vi "Dashboard Main.vi"() -> ()   [LabVIEW 2012]
uses:
  <vilib>/event_ctls.llb/eventvkey.ctl
  <vilib>/Utility/config.llb/Read Key (String).vi
  <vilib>/Utility/config.llb/Read Key (I32).vi
  <vilib>/Utility/config.llb/Write Key (String).vi
  <vilib>/Utility/config.llb/Write Key (I32).vi
  <vilib>/Utility/config.llb/NI_LVConfig.lvlib
panel:
  in  "Camera Enable":bool
  in  "Camera Settings":T1={"Frate Rate"=30, "Compression"=30, "Size"=1} {"Frate Rate" scale=1.0..30.0; "Size" items=["640x480", "320x240", "160x120"]}
  out "Mode":T2(ring)=enum."Auto Disabled"
  out "Camera IP":string
  in  "Dashboard Tab":T3(tab)
  out "Desired Elevation":dbl(slide) scale=0.0..46.0
  out "Compressor Status":bool
  out "Manual RPM":dbl
  in  "Auto Fling":bool
  in  "Auto Spin":bool=TRUE
  in  "Auto Tilt":bool=TRUE
  out "Current Elevation":dbl(slide) scale=0.0..46.0
  out "At Speed":bool
  out "Spin":cluster{dbl, dbl}(knob) scale=0.0..5000.0
  out "Prespin":cluster{dbl, dbl}(knob) scale=0.0..5000.0
  in  "Set Front Pyramid Angle":bool
  in  "Set Feeder Station Preset":bool
  in  "Set Auton Shooter Speed":bool
  in  "Set Rear Pyramid Angle":bool
  in  "Set Behind Pyramid Angle":bool
  in  "Record Autonomous":bool
  in  "DB Camera Config":bool
  out "Mbps":dbl format="%#.1g"
  out "Mbps 2":bool
  out "fps":dbl format="%#.1g"
  in  "Calibrate Arm Top":bool
  in  "Calibrate Arm Bottom":bool
  out "JS1 Z":dbl(slide) scale=-1.0..1.0 scale format="%#_2e"
  out "JS2 Z":dbl(slide) scale=-1.0..1.0 scale format="%#_2e"
  out "Joystick 1":cluster{"X":dbl, "Y":dbl}[](graph)
  out "Joystick 2":cluster{"X":dbl, "Y":dbl}[](graph)
  out "JS Buttons 1":T4
  out "JS Buttons 2":T4
  out "MotorSlide4":dbl(slide) scale=-1.0..1.0 scale format="%#_2e"
  out "MotorSlide3":dbl(slide) scale=-1.0..1.0 scale format="%#_2e"
  out "MotorSlide2":dbl(slide) scale=-1.0..1.0 scale format="%#_2e"
  in  "MotorName3":string="Front Left"
  in  "MotorName4":string="Front Right"
  in  "MotorName1":string="Rear Left"
  in  "MotorName2":string="Rear Right"
  out "MotorChart4":dbl(graph)
  out "MotorChart3":dbl(graph)
  out "MotorChart2":dbl(graph)
  out "MotorSlide1":dbl(slide) scale=-1.0..1.0 scale format="%#_2e"
  out "MotorChart1":dbl(graph)
  out "Battery Value":dbl(slide) scale=0.0..14.0 scale format="%#_2e"
  out "Battery":sgl(graph)
  out "Robot IP":string
  in  "Slider":dbl(slide) scale=0.0..100.0 scale format="%#_3g"
  in  "On/Off":bool caption="Solenoid"
  in  "Test Name":u16(ring) items=["Select the test to run...", "Example Test", "-------------------------------", "List of tests is built in robot code.", "Replace with your own automated tests."]
  in  "Test Tree":string(tree)
  in  "Motor":cluster{"Value":dbl, "Enable":bool} {"Value" scale=-1.0..1.0 scale format="%#_3g"}
  out "Progress":T5 {"Test Progress" scale=0.0..100.0}
  in  "Rev/Fwd":cluster{"Forward":bool, "Reverse":bool}
  in  "Ring":u16(ring) items=["Auto", "Fixed indoor", "Fixed outdoor 1", "Fixed outdoor 2", "Fixed fluorescent 1", "Fixed fluorescent 2", "Hold current"]
  in  "Listbox":i32(listbox)
  in  "Viewer":enum32{"Camera Image", "Variables"}(tab)
  out "Image Error Message":string="Timeout in Camera Communications"
  out "Camera Image":T6(plugin-control)
  out "Tree":string(tree)
  # "Drive & Motors"
  # "Robot IP:"
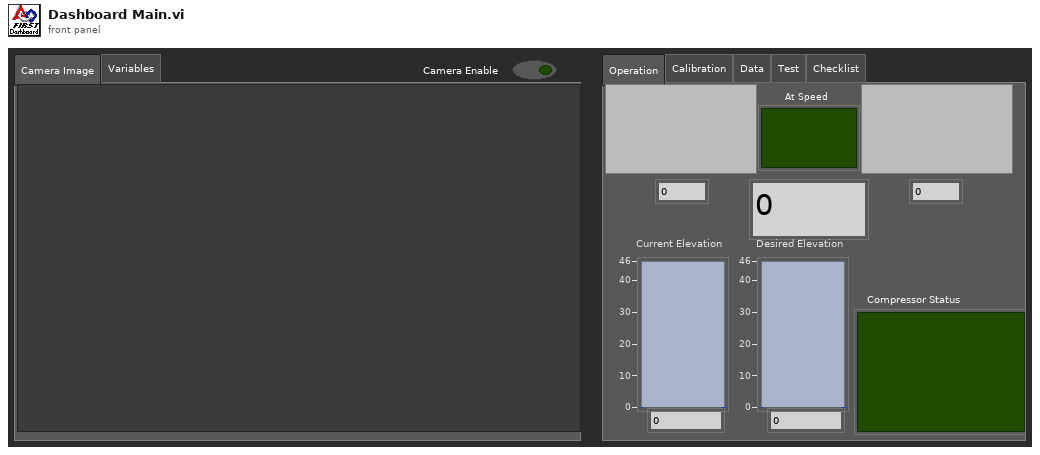
[diagram p1: front panel]
types:
  T1 = cluster{"Frate Rate":i32, "Compression":i32, "Size":u16}
  T2 = enum8{"Tele-Op Disabled", "Tele-Op Enabled", "Auto Disabled", "Auto Enabled", "Test Disabled", "Test Enabled", ""}
  T3 = enum32{"Operation", "Calibration", "Data", "Test", "Checklist"}
  T4 = cluster{bool, bool, bool, bool, bool, bool, bool, bool, bool, bool, bool, bool}
  T5 = cluster{"Test Progress":u8, "Test Progress Text":string}
  T6 = typedef "IMAQ Image.ctl" = refnum<image>
  T7 = typedef "Image Type" = u32
  T8 = typedef "SkeletonTrackState.ctl" = enum32{"NotTracked", "PositionOnly", "Tracked"}
  T9 = cluster{"TrackingState":u8[], "Position":cluster{"x":sgl, "y":sgl, "z":sgl}, cluster{"x":sgl, "y":sgl, "z":sgl, sgl}[], "TrackState":T8}
  T10 = cluster{cluster{"ScaledToPercentRange":dbl, "ScaledToPercentRange":dbl, "ScaledToPercentRange":dbl}, cluster{bool, bool, bool}}[]
  T11 = cluster{cluster{"ScaledToPercentRange":dbl, "ScaledToPercentRange":dbl, "ScaledToPercentRange":dbl}, cluster{bool, bool, bool}}
  T12 = typedef "LVRectTypeDef.ctl" = cluster{"Left":i16, "Top":i16, "Right":i16, "Bottom":i16}
  T13 = cluster{"Competition mode":bool, "Robot Link":bool, "Autonomous":bool, "Enabled":bool, "E-Stop":bool, "Simulated":bool, "TestMode":bool, "Docked Window":bool}
  T14 = cluster{"Boolean Array[0]":bool, "Boolean Array[1]":bool, "Boolean Array[2]":bool, "Boolean Array[3]":bool, "Boolean Array[4]":bool, "Boolean Array[5]":bool, "Boolean Array[6]":bool, "Boolean Array[7]":bool, "Boolean Array[8]":bool, "Boolean Array[9]":bool, "Boolean Array[10]":bool, "Boolean Array[11]":bool}
  T15 = typedef "NI_LVConfig.lvlib/Config Data RefNum.ctl" = refnum<k1>
  T16 = typedef "eventvkey.ctl" = enum16{"ASCII", "Enter", "Return", "Shift", "Ctrl", "Alt", "Cmd", "Opt", "Caps", "NumLock", "Clear", "Break", "Up", "Down", "Left", "Right", "Insert", "Delete", "Home", "End", "PageUp", "PageDown", "Escape", "Help", "Pause", "ScrollLock", "F1", "F2", "F3", "F4", "F5", "F6", "F7", "F8", "F9", "F10", "F11", "F12", "F13", "F14", "F15", "F16", "F17", "F18", "F19", "F20", "F21", "F22", "F23", "F24", "Play", "VolumeUp", "VolumeDown", "Mute", "Two Byte Char"}
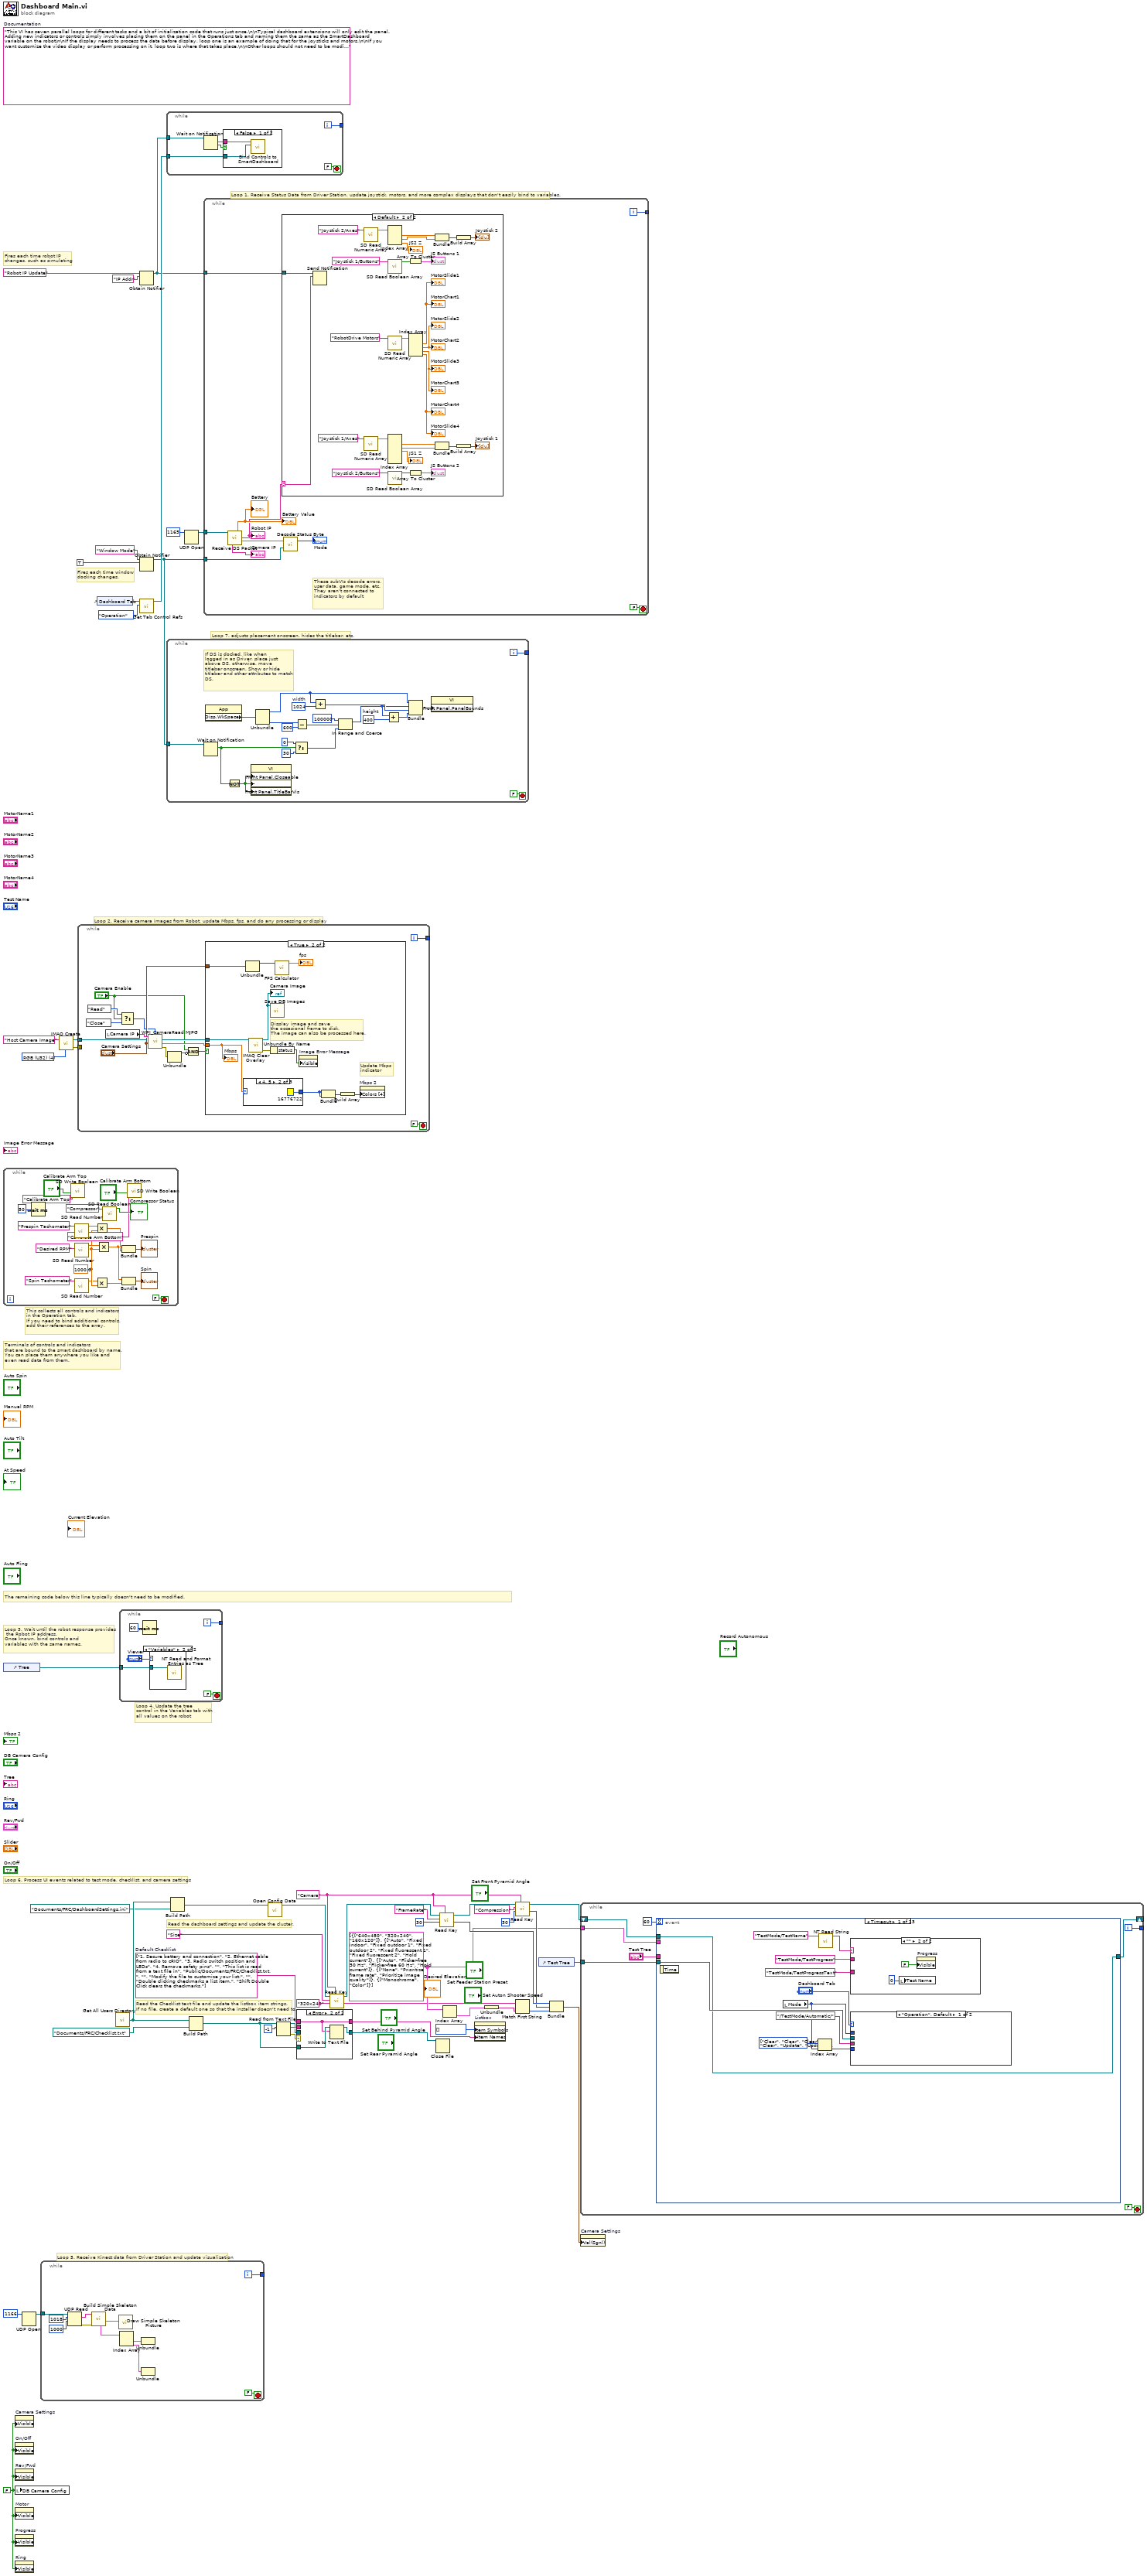
[diagram p0: block diagram]
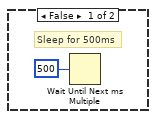
[diagram p3: hidden frame]
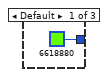
[diagram p4: hidden frame]
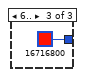
[diagram p5: hidden frame]
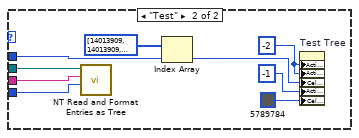
[diagram p7: hidden frame]
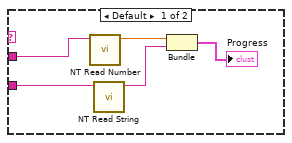
[diagram p8: hidden frame]
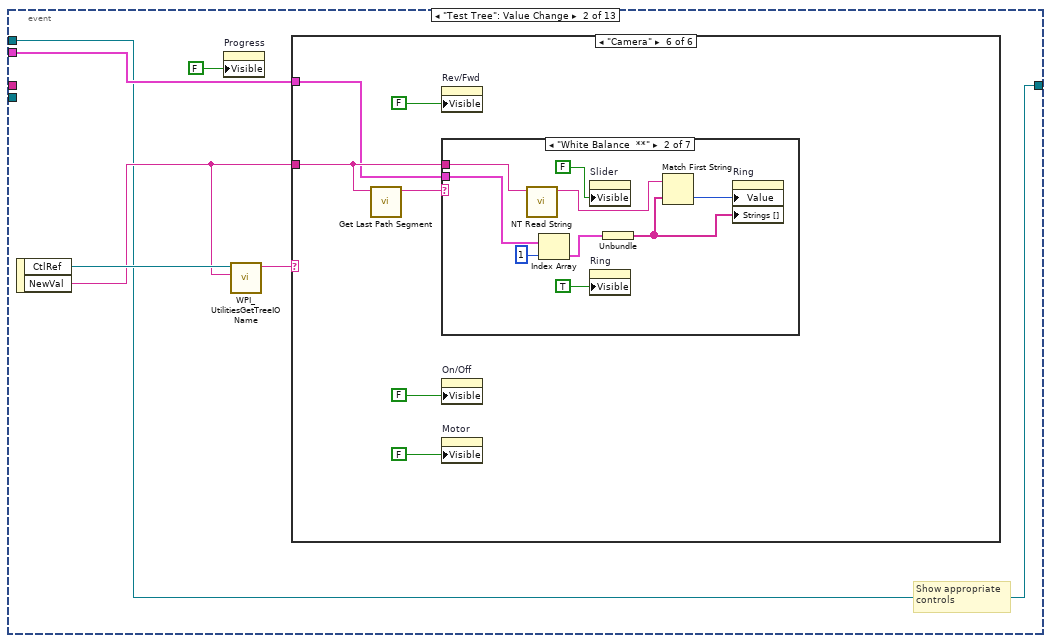
[diagram p9: hidden frame]
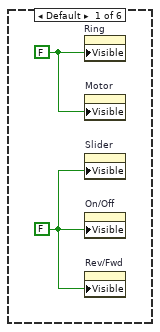
[diagram p10: hidden frame]
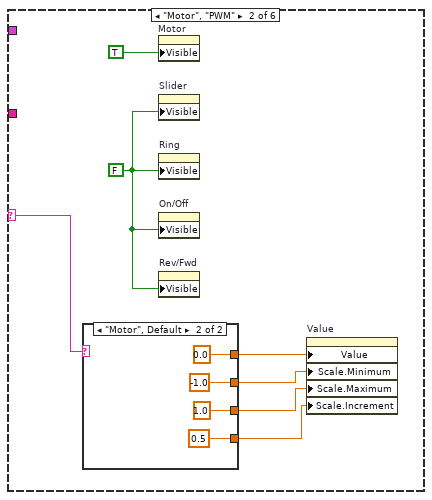
[diagram p11: hidden frame]
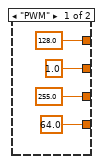
[diagram p12: hidden frame]
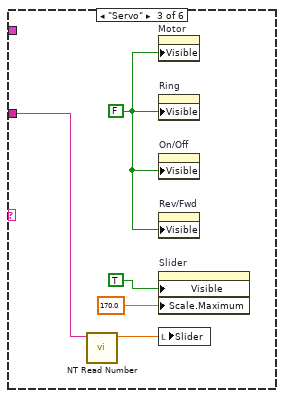
[diagram p13: hidden frame]
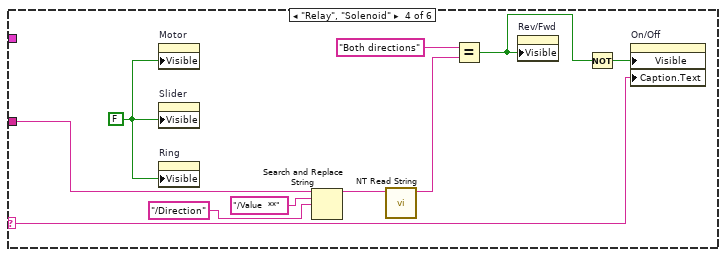
[diagram p14: hidden frame]
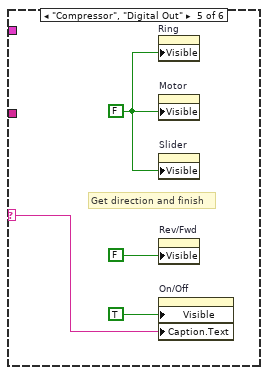
[diagram p15: hidden frame]
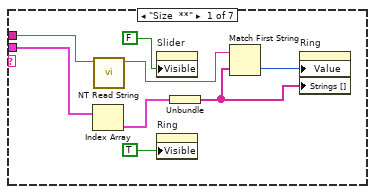
[diagram p16: hidden frame]
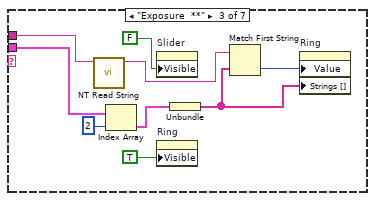
[diagram p17: hidden frame]
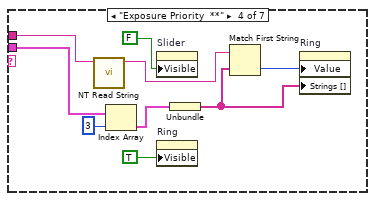
[diagram p18: hidden frame]
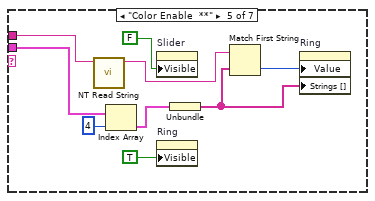
[diagram p19: hidden frame]
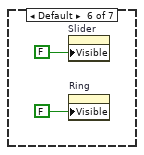
[diagram p20: hidden frame]
diagram:
  w21 = "Camera"
  w13 = cluster{string[]}[] [{["640x480", "320x240", "160x120"]}, {["Auto", "Fixed indoor", "Fixed outdoor 1", "Fixed outdoor 2", "Fixed fluorescent 1", "Fixed fluorescent 2", "Hold current"]}, {["Auto", "Flicker-free 50 Hz", "Flicker-free 60 Hz", "Hold current"]}, {["None", "Prioritize frame rate", "Prioritize image quality"]}, {["Monochrome", "Color"]}]
  w29 = string[] ["1. Secure battery and connection", "2. Ethernet cable from radio to cRIO", "3. Radio switch position and LEDs", "4. Remove safety pins", "", "This list is read from a text file in", "Public/Documents/FRC/Checklist.txt.", "", "Modify the file to customize your list.", "", "Double clicking checkmarks a list item.", "Shift Double Click clears the checkmarks."]  # Default Checklist
  w27 = FALSE ("Visible")
  (unwired) "This VI has seven parallel loops for different tasks and a bit of initialization code that runs just once.\n\nTypical dashboard extensions will only edit the panel. Adding new indicators or controls simply involves placing them on the panel in the Operations tab and naming them the same as the SmartDashboard variable on the robot\n\nIf the display needs to process the data before display, loop one is an example of doing that for the joysticks and motors.\n\nIf you want customize the video display or perform processing on it, loop two is where that takes place.\n\nOther loops should not need to be modified. They are pretty standard, and document the task they perform."  # Documentation
  w50 = T7 4 items=["Grayscale (U8)", "Grayscale (I16)", "Grayscale (SGL)", "Complex (CSG)", "RGB (U32)", "HSL (U32)", "RGB (U64)"] ("Image Type")
  # "Fires each time robot IP\nchanges, such as simulating"
  # "Fires each time window\ndocking changes."
  # "Read the Checklist text file and update the listbox item strings.\nIf no file, create a default one so that the installer doesn't need to."
  # "This collects all controls and indicators\nin the Operation tab.\nIf you need to bind additional controls,\nadd their references to the array."
  # "The remaining code below this line typically doesn't need to be modified."
  # "Loop 6. Process UI events related to test mode, checklist, and camera settings"
  # "Read the dashboard settings and update the cluster."
  # "Terminals of controls and indicators\nthat are bound to the smart dashboard by name.\nYou can place them anywhere you like and\neven read data from them."
  # "Loop 4. Update the tree\ncontrol in the Variables tab with\nall values on the robot"
  # "Loop 3. Wait until the robot response provides\n the Robot IP address.\nOnce known, bind controls and\nvariables with the same names."
  # "Loop 5. Receive Kinect data from Driver Station and update visualization"
  # "Loop 7. adjusts placement onscreen, hides the titlebar, etc."
  # "Loop 1. Receive Status Data from Driver Station, update joystick, motors, and more complex displays that don't easily bind to variables."
  # "Loop 2. Receive camera images from Robot, update Mbps, fps, and do any processing or display"
  n1 = while {
    stop <- FALSE stop-if-true
    w65 = 1000.0 ("y")
    n2 = Wait (ms)(milliseconds to wait=u32 50) -> ()  [unwired: 1 out]
    n3 = call <vilib>:"SD Write Boolean.vi"("Boolean"="Calibrate Arm Top", "Name"="Calibrate Arm Top") -> ()  [unwired: 8 in, 2 out]
    n4 = call <vilib>:"SD Read Number.vi"("Name"="Prespin Tachometer") -> ("Numeric"=w64:dbl)  [unwired: 8 in, 2 out]
    n5 = call <vilib>:"SD Read Number.vi"("Table Prefix"="Desired RPM") -> ("Numeric"=w66:dbl)  [unwired: 8 in, 2 out]
    n6 = call <vilib>:"SD Read Number.vi"("Name"="Spin Tachometer") -> ("Numeric"=w62:dbl)  [unwired: 8 in, 2 out]
    n7 = Multiply(x=w64, y=w65) -> (x*y=w63:dbl)
    n8 = Multiply(x=w62, y=w65) -> (x*y=w61:dbl)
    n9 = Multiply(x=w66, y=w65) -> (x*y=w67:dbl)
    n10 = call <vilib>:"SD Read Boolean.vi"("Name"="Compressor") -> ("Boolean"=→"Compressor Status":bool)  [unwired: 8 in, 2 out]
    n11 = Bundle(w67, w63) -> (→"Prespin":cluster{dbl, dbl})  [unwired: 1 in]
    n12 = Bundle(w67, w61) -> (→"Spin":cluster{dbl, dbl})  [unwired: 1 in]
    n13 = call <vilib>:"SD Write Boolean.vi"("Boolean"="Calibrate Arm Bottom", "Name"="Calibrate Arm Bottom") -> ()  [unwired: 8 in, 2 out]
  }
  n14 = control-ref of="Tree"() -> (w2:refnum<vi>)
  n15 = property on="Camera Settings" class="Clust (strict)"("Visible"=w27) -> ()  [unwired: 2 in, 2 out]
  n16 = property on="On/Off" class="Bool (strict)"("Visible"=w27) -> ()  [unwired: 2 in, 2 out]
  n17 = property on="Rev/Fwd" class="Clust (strict)"("Visible"=w27) -> ()  [unwired: 2 in, 2 out]
  n18 = local write "DB Camera Config"(w27) -> ()
  n19 = property on="Motor" class="Clust (strict)"("Visible"=w27) -> ()  [unwired: 2 in, 2 out]
  n20 = property on="Progress" class="Clust (strict)"("Visible"=w27) -> ()  [unwired: 2 in, 2 out]
  n21 = property on="Ring" class="Ring (strict)"("Visible"=w27) -> ()  [unwired: 2 in, 2 out]
  n22 = UDP Open(11:u16 1166 ("port")) -> (port=w45:refnum<k16>)  [unwired: 2 in, 4 out]
  n23 = while {
    tunnel: w45 -> [w81]
    tunnel: [w74] -> _
    i -> [w74]
    stop <- FALSE stop-if-true
    n24 = UDP Read(connection ID=w81, max size (548)=1018 ("bytes to read"), timeout ms (25000)=1000) -> (data out=w79:string, error out=w73:errorcluster)  [unwired: 1 in, 3 out]
    n25 = call "Build Simple Skeleton Data.vi"("error in (no error)"=w73, "data in"=w79) -> ("Skeleton Data"=w80:T9, "Simple Joystick Info"=w77:T10)  [unwired: 5 in, 3 out]
    n26 = call "Draw Simple Skeleton Picture.vi"("Simple Skeleton"=w80) -> ()  [unwired: 10 in, 1 out]
    n27 = Index Array(array=w77) -> (element #1=w76:T11, element #2=w75:T11)  [unwired: 2 in]
    n28 = Unbundle(w76) -> ()  [unwired: 2 out]
    n29 = Unbundle(w75) -> ()  [unwired: 2 out]
  }
  n30 = call "IMAQ Create"("Image Name"="Host Camera Image", "Image Type"=w50) -> ("New Image"=w48:T6, "error out"=w47:errorcluster)  [unwired: 2 in, 1 out]
  n31 = while {
    tunnel: w48 -> [w93]
    tunnel: w47 -> [_]
    tunnel: [w96] -> _
    i -> [w96]
    stop <- FALSE stop-if-true
    n32 = local read "Camera IP"() -> (w95:string)
    n33 = Select(t=enum16{"Read", "Reopen", "Close"}."Read" ("Operation"), s="Camera Enable", f=enum16{"Read", "Reopen", "Close"}."Close" ("Operation")) -> (s? t:f=w88:enum16{"Read", "Reopen", "Close"})
    n34 = call <vilib>:"WPI_CameraRead MJPG.vi"("Operation"=w88, "Camera Settings"="Camera Settings", "Image"=w93, "address"=w95) -> ("error out"=w87:errorcluster, "Bandwidth (kbps)"=w91:dbl, "Image Out"=w92:T6)  [unwired: 5 in]
    n35 = Unbundle(w87) -> ("status"=w85:bool)  [unwired: 2 out]
    n36 = Compound Arithmetic op=AND("Camera Enable", invert w85) -> (w84:bool)
    n37 = case shown="True" w84 {
      tunnel: "Camera Settings" -> [_ w100]
      tunnel: w92 -> [_ w103]
      tunnel: w91 -> [_ w102]
      frame False {
        # "Sleep for 500ms"
        n38 = Wait Until Next ms Multiple(millisecond multiple=u32 500) -> ()  [unwired: 1 out]
      }
      frame True {
        # "Display image and save\nthe occasional frame to disk.\nThe image can also be processed here."
        # "Update Mbps\nindicator"
        n39 = case shown="4, 5" w102 {
          tunnel: [u32 6618880 ("Color Box") u32 16776722 ("Color Box") u32 16716800 ("Color Box")] -> w104
          frame Default {
          }
          frame 4, 5 {
          }
          frame 6.. {
          }
        }
        n40 = Unbundle(w100) -> ("Frate Rate"=w99:i32)  [unwired: 2 out]
        n41 = call "IMAQ Clear Overlay"("Image"=w103) -> ("error out"=w108:errorcluster, "Image Out"=w107:T6)  [unwired: 2 in, 7 out]
        "Camera Image" <- w107
        n42 = call "Save DB Images.vi"("Image"=w107) -> ()  [unwired: 2 in, 1 out]
        n43 = Unbundle By Name(w108) -> ("status"=w109:bool)
        n44 = call "FPS Calculator.vi"("Average Count"=w99) -> ("fps"=→"fps":dbl)  [unwired: 10 in]
        n45 = property on="Image Error Message" class="Str"("Visible"=w109) -> ()  [unwired: 2 in, 2 out]
        n46 = Bundle("Color Box"=w104, "Color Box"=w104) -> (w106:cluster{"Color Box":u32, "Color Box":u32})  [unwired: 1 out]
        n47 = Build Array(w106) -> (w105:cluster{"Color Box":u32, "Color Box":u32}[])
        n48 = property on="Mbps 2" class="Bool (strict)"("Colors [4]"=w105) -> ()  [unwired: 2 in, 2 out]
        "Mbps" <- w102
      }
    }
  }
  n49 = control-ref of="Dashboard Tab"() -> (w43:refnum<vi>)
  n50 = call "Get All Users Directory.vi"() -> ("All User Path"=w26:path)
  n51 = while {
    tunnel: [w114] -> _
    tunnel: w2 -> [w113]
    i -> [w114]
    stop <- FALSE stop-if-true
    n52 = Wait (ms)(milliseconds to wait=u32 60) -> ()  [unwired: 1 out]
    n53 = case shown="\"Variables\"" "Viewer" {
      tunnel: w113 -> [_ w118]
      frame Default {
      }
      frame "Variables" {
        n54 = call <vilib>:"NT Read and Format Entries as Tree.vi"("Tree Refnum"=w118) -> ()  [unwired: 9 in, 2 out]
      }
    }
  }
  n55 = Obtain Notifier(name (unnamed)="Robot IP Update", notification data type="IP Addr" ("name (unnamed)")) -> (notifier out=w40:refnum<notifier>)  [unwired: 2 in, 2 out]
  n56 = Obtain Notifier(name (unnamed)="Window Mode", notification data type=TRUE) -> (notifier out=w33:refnum<notifier>)  [unwired: 2 in, 2 out]
  n57 = call <vilib>:"Get Tab Control Refs.vi"("Page Index"=enum32{"Operation", "Test"}."Operation" ("Dashboard Tab"), "TabControl in"=w43) -> ("ControlsOnPage"=w44:refnum<vi>[])  [unwired: 9 in]
  n58 = while {
    tunnel: w44 -> [w124]
    tunnel: w40 -> [w121]
    tunnel: [w119] -> _
    i -> [w119]
    stop <- FALSE stop-if-true
    n59 = Wait on Notification(notifier=w121) -> (notification=w120:string, timed out?=w122:bool)  [unwired: 3 in, 2 out]
    n60 = case shown="False" w122 {
      tunnel: w124 -> [w126 _]
      tunnel: w120 -> [w125 _]
      frame False {
        n61 = call <vilib>:"Bind Controls to SmartDashboard.vi"("Bound Control Refs"=w126, "Server IP Address"=w125) -> ()  [unwired: 10 in]
      }
      frame True {
      }
    }
  }
  n62 = while {
    tunnel: w33 -> [w145]
    tunnel: [w143] -> _
    i -> [w143]
    stop <- FALSE stop-if-true
    w135 = 1024  # width
    w138 = 400  # height
    # "If DS is docked, like when\nlogged in as Driver, place just\nabove DS, otherwise, move\ntitlebar onscreen. Show or hide\ntitlebar and other attributes to match\nDS."
    n63 = Wait on Notification(notifier=w145) -> (notification=w130:bool)  [unwired: 3 in, 3 out]
    n64 = property class="App"() -> ("Disp.WkSpace"=w141:T12)  [unwired: 2 in, 2 out]
    n65 = Not(x=w130) -> (.not. x?=w144:bool)
    n66 = property class="VI"("Front Panel.Closeable"=w144, "Front Panel.Minimizeable"=w144, "Front Panel.TitleBarVis"=w144) -> ()  [unwired: 2 in, 2 out]
    n67 = Unbundle(w141) -> ("Left"=w139:i16, "Bottom"=w136:i16)  [unwired: 2 out]
    n68 = Select(t=0, s=w130, f=30) -> (s? t:f=w129:i32)
    n69 = Subtract(x=w136, y=600) -> (x-y=w133:i32)
    n70 = Add(x=w139, y=w135) -> (x+y=w140:i32)
    n71 = In Range and Coerce(upper limit=100000, x=w133, lower limit=w129) -> (coerced(x)=w127:i32)  [unwired: 1 out]
    n72 = Add(x=w127, y=w138) -> (x+y=w137:i32)
    n73 = Bundle("Left"=w139, w127, w140, w137) -> (w142:cluster{"Left":i16, i32, i32, i32})  [unwired: 1 out]
    n74 = property class="VI"("Front Panel.PanelBounds"=w142) -> ()  [unwired: 2 in, 2 out]
  }
  n75 = Build Path(base path=w26, name or relative path=path "Documents/FRC/DashboardSettings.ini") -> (appended path=w25:path)
  n76 = UDP Open(11:u16 1165 ("port")) -> (port=w51:refnum<k16>)  [unwired: 2 in, 4 out]
  n77 = Build Path(base path=w26, name or relative path=path "Documents/FRC/Checklist.txt") -> (appended path=w30:path)
  n78 = while {
    tunnel: w51 -> [w154]
    tunnel: w40 -> [w148]
    tunnel: w33 -> [w152]
    tunnel: [w149] -> _
    i -> [w149]
    stop <- FALSE stop-if-true
    # "These subVIs decode errors, user data, game mode, etc.\nThey aren't connected to indicators by default"
    n79 = call "Receive DS Packet.vi"("Recv Socket"=w154) -> ("Battery"=→"Battery" →"Battery Value":sgl, "Robot IP Address"=w147:string, "Status"=w155:T13, "Camera IP Address"=→"Camera IP":string)  [unwired: 1 in, 10 out]
    "Robot IP" <- w147
    n80 = case shown="Default" w147 {
      selector: w147 -> [_ w157]
      tunnel: w148 -> [_ w158]
      frame "0.0.0.0" {
        # "Robot not responding, don't poll the variables"
      }
      frame Default {
        n81 = Send Notification(notification=w157, notifier=w158) -> ()  [unwired: 1 in, 2 out]
        n82 = call <vilib>:"SD Read Numeric Array.vi"("Name"="Joystick 2/Axes") -> ("Numeric Array"=w168:dbl[])  [unwired: 8 in, 2 out]
        n83 = call <vilib>:"SD Read Numeric Array.vi"("Name"="Joystick 1/Axes") -> ("Numeric Array"=w174:dbl[])  [unwired: 8 in, 2 out]
        n84 = Index Array(array=w168) -> (element #1=w163:dbl, element #2=w162:dbl, element #3=→"JS2 Z":dbl)  [unwired: 3 in]
        n85 = call <vilib>:"SD Read Boolean Array.vi"("Name"="Joystick 1/Buttons") -> ("Boolean Array"=w176:bool[])  [unwired: 8 in, 2 out]
        n86 = call <vilib>:"SD Read Numeric Array.vi"("Name"="RobotDrive Motors") -> ("Numeric Array"=w181:dbl[])  [unwired: 8 in, 2 out]
        n87 = Index Array(array=w174) -> (element #1=w171:dbl, element #2=w172:dbl, element #3=→"JS1 Z":dbl)  [unwired: 6 in, 3 out]
        n88 = call <vilib>:"SD Read Boolean Array.vi"("Name"="Joystick 2/Buttons") -> ("Boolean Array"=w167:bool[])  [unwired: 8 in, 2 out]
        n89 = Array To Cluster(array=w176) -> (cluster=→"JS Buttons 1":T14)
        n90 = Array To Cluster(array=w167) -> (cluster=→"JS Buttons 2":T14)
        n91 = Index Array(array=w181) -> (element #1=→"MotorChart1" →"MotorSlide1":dbl, element #2=→"MotorSlide2" →"MotorChart2":dbl, element #3=→"MotorChart3" →"MotorSlide3":dbl, element #4=→"MotorChart4" →"MotorSlide4":dbl)  [unwired: 4 in]
        n92 = Bundle("Numeric"=w163, "Numeric"=w162) -> (w164:cluster{"Numeric":dbl, "Numeric":dbl})  [unwired: 1 in]
        n93 = Bundle("Numeric"=w171, "Numeric"=w172) -> (w170:cluster{"Numeric":dbl, "Numeric":dbl})  [unwired: 1 in]
        n94 = Build Array(w164) -> (→"Joystick 2":cluster{"Numeric":dbl, "Numeric":dbl}[])
        n95 = Build Array(w170) -> (→"Joystick 1":cluster{"Numeric":dbl, "Numeric":dbl}[])
      }
    }
    n96 = call "Decode Status Byte.vi"("Window Mode Notifier"=w152, "Status"=w155) -> ("Mode"=→"Mode":T2)  [unwired: 1 out]
  }
  n97 = call <vilib>:"Open Config Data.vi"("configuration file path"=w25) -> ("refnum"=w24:T15)  [unwired: 8 in, 2 out]
  n98 = Read from Text File(file (use dialog)=w30, count=-1 ("timeout ms (25000)")) -> (refnum out=w8:refnum<file>, text=w31:string[], error out=w32:errorcluster)  [unwired: 2 in, 1 out]
  n99 = case shown="Error" w32 {
    tunnel: w31 -> [w186 _]
    tunnel: [w186 w188] -> w28
    tunnel: w29 -> [_ w188]
    tunnel: w30 -> [_ w189]
    tunnel: [w185 w187] -> w7
    tunnel: w8 -> [w185 _]
    frame No Error {
    }
    frame Error {
      n100 = Write to Text File(file (use dialog)=w189, text=w188) -> (refnum out=w187:refnum<file>)  [unwired: 2 in, 2 out]
    }
  }
  n101 = call-poly <vilib>:"Read Key.vi"("section"=w21, "default value"="320x240", "key"="Size", "refnum"=w24) -> ("value"=w11:string, "refnum out"=w6:T15)  [unwired: 2 in, 4 out]
  n102 = Close File(refnum=w7) -> ()  [unwired: 1 in, 2 out]
  n103 = call-poly <vilib>:"Read Key.vi"("section"=w21, "default value"=30, "key"="FrameRate", "refnum"=w6) -> ("value"=w16:i32, "refnum out"=w5:T15)  [unwired: 1 in, 5 out]
  n104 = Index Array(array=w13) -> (element=w14:cluster{string[]})  [unwired: 1 in]
  n105 = property on="Listbox" class="LstBox (strict)"("Item Symbols"=i32[] [], "Item Names"=w28) -> ()  [unwired: 2 in, 2 out]
  n106 = Unbundle(w14) -> (w12:string[])
  n107 = call-poly <vilib>:"Read Key.vi"("section"=w21, "default value"=30, "key"="Compression", "refnum"=w5) -> ("value"=w15:i32, "refnum out"=w3:T15)  [unwired: 1 in, 5 out]
  n108 = Match First String(2:w12, 3:w11) -> (0:w10:i32)  [unwired: 1 out]
  n109 = control-ref of="Test Tree"() -> (w1:refnum<vi>)
  n110 = Bundle("value"=w16, "value"=w15, "index"=w10) -> (w4:cluster{"value":i32, "value":i32, "index":i32})  [unwired: 1 out]
  n111 = while {
    tunnel: w13 -> [w194]
    shift-right: [w193] -> _
    shift-left: w3 -> [w192]
    tunnel: [w191] -> _
    tunnel: w1 -> [w190]
    i -> [w191]
    stop <- FALSE stop-if-true
    n112 = event shown="[0] Timeout" {
      selector: _ -> [_ _ _ _ _ _ _ _ _ _ _ _ _]
      dyn-events: _ -> [_ _ _ _ _ _ _ _ _ _ _ _ _]
      timeout: u32 60 ("milliseconds to wait") -> [_ _ _ _ _ _ _ _ _ _ _ _ _]
      tunnel: w190 -> [w204 _ _ _ _ _ _ _ _ _ _ _ _]
      tunnel: "Test Tree" -> [_ _ _ _ _ _ _ _ w398 w406 w408 w412 w420]
      tunnel: w194 -> [_ w226 _ _ _ _ w362 w392 _ _ _ _ _]
      tunnel: [w198 w225 _ w328 w336 w348 w361 w385 w397 w404 w407 w411 w419] -> w193
      tunnel: w192 -> [w198 w225 _ w328 w336 w348 w360 w385 w397 w404 w407 w411 w419]
      event Timeout {
        w203 = enum16{"Update", "Clear"}[] [enum."Clear", enum."Clear", enum."Clear", enum."Clear", enum."Update", enum."Update", enum."Clear"] items=["Update", "Clear"]
        n113 = event-data() -> ()  [unwired: 1 in, 1 out]
        n114 = local read "Mode"() -> (w201:T2)
        n115 = Index Array(array=w203, index=w201) -> (element=w202:enum16{"Update", "Clear"})
        n116 = call <vilib>:"NT Read String.vi"("Name"="TestMode/TestName") -> ("String"=w207:string)  [unwired: 9 in, 1 out]
        n117 = case shown="\"\"" w207 {
          tunnel: "TestMode/TestProgress" ("Name") -> [w219 _]
          tunnel: "TestMode/TestProgressText" ("Name") -> [w218 _]
          frame Default {
            n118 = call <vilib>:"NT Read Number.vi"("Name"=w219) -> ("Numeric"=w220:dbl)  [unwired: 9 in, 1 out]
            n119 = call <vilib>:"NT Read String.vi"("Name"=w218) -> ("String"=w221:string)  [unwired: 9 in, 1 out]
            n120 = Bundle("Numeric"=w220, "String"=w221) -> (→"Progress":cluster{"Numeric":dbl, "String":string})  [unwired: 1 in]
          }
          frame "" {
            n121 = local write "Test Name"(u16 0) -> ()
            n122 = property on="Progress" class="Clust (strict)"("Visible"=FALSE) -> ()  [unwired: 2 in, 2 out]
          }
        }
        n123 = case shown="\"Operation\", Default" "Dashboard Tab" {
          tunnel: w204 -> [_ w217]
          tunnel: "/TestMode/Automatic/" ("Name Pattern") -> [_ w216]
          tunnel: w202 -> [_ w215]
          tunnel: w201 -> [_ w213]
          frame "Operation", Default {
          }
          frame "Test" {
            w212 = -2 ("Active Item:Row Number")
            n124 = call <vilib>:"NT Read and Format Entries as Tree.vi"("Operation"=w215, "Name Pattern"=w216, "Tree Refnum"=w217) -> ()  [unwired: 7 in, 2 out]
            n125 = Index Array(array=u32[] [14013909, 14013909, 14013909, 14013909, 14013909, 16777215, 14013909], index=w213) -> (element=w211:u32)
            n126 = property on="Test Tree" class="Tree (strict)"("Active Item Row Number"=w212, "ActiveColNum"=w212, "CellBG"=w211, "Active Item Row Number"=-1 ("Active Item:Row Number"), "CellBG"=u32 5789784 ("Color Box")) -> ()  [unwired: 2 in, 2 out]
          }
        }
      }
      event "Test Tree": Value Change {
        # "Show appropriate\ncontrols"
        n127 = event-data() -> ("CtlRef"=w229:refnum<vi>, "NewVal"=w227:string)  [unwired: 1 in]
        n128 = property on="Progress" class="Clust (strict)"("Visible"=FALSE) -> ()  [unwired: 2 in, 2 out]
        n129 = call <vilib>:"WPI_UtilitiesGetTreeIOName.vi"("NewVal"=w227, "TreeControl in"=w229) -> ("I/O Name"=w230:string)  [unwired: 9 in]
        n130 = case shown="\"Camera\"" w230 {
          selector: w230 -> [_ w237 _ w255 w264 _]
          tunnel: w227 -> [_ _ w252 w254 _ w271]
          tunnel: w226 -> [_ _ _ _ _ w270]
          frame Default {
            w232 = FALSE ("Visible")
            w231 = FALSE ("Visible")
            n131 = property on="Ring" class="Ring (strict)"("Visible"=w231) -> ()  [unwired: 2 in, 2 out]
            n132 = property on="Motor" class="Clust (strict)"("Visible"=w231) -> ()  [unwired: 2 in, 2 out]
            n133 = property on="Slider" class="Slide (strict)"("Visible"=w232) -> ()  [unwired: 2 in, 2 out]
            n134 = property on="On/Off" class="Bool (strict)"("Visible"=w232) -> ()  [unwired: 2 in, 2 out]
            n135 = property on="Rev/Fwd" class="Clust (strict)"("Visible"=w232) -> ()  [unwired: 2 in, 2 out]
          }
          frame "Motor", "PWM" {
            w238 = FALSE ("Visible")
            n136 = case shown="\"Motor\", Default" w237 {
              tunnel: [1.0 ("Value") -1.0 ("Value")] -> w236
              tunnel: [255.0 ("Value") 1.0 ("Value")] -> w235
              tunnel: [128.0 ("Value") 0.0 ("Value")] -> w234
              tunnel: [64.0 ("Value") 0.5 ("Value")] -> w233
              frame "PWM" {
              }
              frame "Motor", Default {
              }
            }
            n137 = property on="Motor" class="Clust (strict)"("Visible"=TRUE) -> ()  [unwired: 2 in, 2 out]
            n138 = property on="Slider" class="Slide (strict)"("Visible"=w238) -> ()  [unwired: 2 in, 2 out]
            n139 = property on="Ring" class="Ring (strict)"("Visible"=w238) -> ()  [unwired: 2 in, 2 out]
            n140 = property on="On/Off" class="Bool (strict)"("Visible"=w238) -> ()  [unwired: 2 in, 2 out]
            n141 = property on="Rev/Fwd" class="Clust (strict)"("Visible"=w238) -> ()  [unwired: 2 in, 2 out]
            n142 = property on="Value" class="Slide (strict)"("Value"=w234, "Scale.Minimum"=w236, "Scale.Maximum"=w235, "Scale.Increment"=w233) -> ()  [unwired: 2 in, 2 out]
          }
          frame "Servo" {
            w250 = FALSE ("Visible")
            n143 = call <vilib>:"NT Read Number.vi"("Name"=w252) -> ("Numeric"=w251:dbl)  [unwired: 9 in, 1 out]
            n144 = property on="Motor" class="Clust (strict)"("Visible"=w250) -> ()  [unwired: 2 in, 2 out]
            n145 = property on="Ring" class="Ring (strict)"("Visible"=w250) -> ()  [unwired: 2 in, 2 out]
            n146 = property on="On/Off" class="Bool (strict)"("Visible"=w250) -> ()  [unwired: 2 in, 2 out]
            n147 = property on="Rev/Fwd" class="Clust (strict)"("Visible"=w250) -> ()  [unwired: 2 in, 2 out]
            n148 = property on="Slider" class="Slide (strict)"("Visible"=TRUE, "Scale.Maximum"=170.0 ("Scale.Range:Maximum")) -> ()  [unwired: 2 in, 2 out]
            n149 = local write "Slider"(w251) -> ()
          }
          frame "Relay", "Solenoid" {
            w253 = FALSE ("Visible")
            n150 = property on="Motor" class="Clust (strict)"("Visible"=w253) -> ()  [unwired: 2 in, 2 out]
            n151 = property on="Slider" class="Slide (strict)"("Visible"=w253) -> ()  [unwired: 2 in, 2 out]
            n152 = property on="Ring" class="Ring (strict)"("Visible"=w253) -> ()  [unwired: 2 in, 2 out]
            n153 = Search and Replace String(input string=w254, search string="/Value  **", replace string="/Direction") -> (result string=w260:string)  [unwired: 5 in, 3 out]
            n154 = call <vilib>:"NT Read String.vi"("Name"=w260) -> ("String"=w258:string)  [unwired: 9 in, 1 out]
            n155 = Equal?(x="Both directions", y=w258) -> (x = y?=w256:bool)
            n156 = property on="Rev/Fwd" class="Clust (strict)"("Visible"=w256) -> ()  [unwired: 2 in, 2 out]
            n157 = Not(x=w256) -> (.not. x?=w257:bool)
            n158 = property on="On/Off" class="Bool (strict)"("Visible"=w257, "Caption.Text"=w255) -> ()  [unwired: 2 in, 2 out]
          }
          frame "Compressor", "Digital Out" {
            w263 = FALSE ("Visible")
            # "Get direction and finish"
            n159 = property on="Ring" class="Ring (strict)"("Visible"=w263) -> ()  [unwired: 2 in, 2 out]
            n160 = property on="Motor" class="Clust (strict)"("Visible"=w263) -> ()  [unwired: 2 in, 2 out]
            n161 = property on="Slider" class="Slide (strict)"("Visible"=w263) -> ()  [unwired: 2 in, 2 out]
            n162 = property on="Rev/Fwd" class="Clust (strict)"("Visible"=FALSE) -> ()  [unwired: 2 in, 2 out]
            n163 = property on="On/Off" class="Bool (strict)"("Visible"=TRUE, "Caption.Text"=w264) -> ()  [unwired: 2 in, 2 out]
          }
          frame "Camera" {
            n164 = call <vilib>:"Get Last Path Segment.vi"("String in"=w271) -> ("String out"=w272:string)  [unwired: 10 in]
            n165 = property on="Rev/Fwd" class="Clust (strict)"("Visible"=FALSE) -> ()  [unwired: 2 in, 2 out]
            n166 = case shown="\"White Balance  **\"" w272 {
              tunnel: w271 -> [w278 w287 w296 w305 w314 _ w320]
              tunnel: w270 -> [w276 w284 w293 w302 w311 _ _]
              frame "Size  **" {
                n167 = Index Array(array=w276) -> (element=w275:cluster{string[]})  [unwired: 1 in]
                n168 = call <vilib>:"NT Read String.vi"("Name"=w278) -> ("String"=w277:string)  [unwired: 9 in, 1 out]
                n169 = property on="Slider" class="Slide (strict)"("Visible"=FALSE) -> ()  [unwired: 2 in, 2 out]
                n170 = property on="Ring" class="Ring (strict)"("Visible"=TRUE) -> ()  [unwired: 2 in, 2 out]
                n171 = Unbundle(w275) -> (w273:string[])
                n172 = Match First String(2:w273, 3:w277) -> (0:w274:i32)  [unwired: 1 out]
                n173 = property on="Ring" class="Ring (strict)"("Value"=w274, "Strings []"=w273) -> ()  [unwired: 2 in, 2 out]
              }
              frame "White Balance  **" {
                n174 = call <vilib>:"NT Read String.vi"("Name"=w287) -> ("String"=w286:string)  [unwired: 9 in, 1 out]
                n175 = Index Array(array=w284, index=1) -> (element=w285:cluster{string[]})
                n176 = property on="Slider" class="Slide (strict)"("Visible"=FALSE) -> ()  [unwired: 2 in, 2 out]
                n177 = property on="Ring" class="Ring (strict)"("Visible"=TRUE) -> ()  [unwired: 2 in, 2 out]
                n178 = Unbundle(w285) -> (w282:string[])
                n179 = Match First String(2:w282, 3:w286) -> (0:w281:i32)  [unwired: 1 out]
                n180 = property on="Ring" class="Ring (strict)"("Value"=w281, "Strings []"=w282) -> ()  [unwired: 2 in, 2 out]
              }
              frame "Exposure  **" {
                n181 = call <vilib>:"NT Read String.vi"("Name"=w296) -> ("String"=w295:string)  [unwired: 9 in, 1 out]
                n182 = Index Array(array=w293, index=2) -> (element=w294:cluster{string[]})
                n183 = property on="Slider" class="Slide (strict)"("Visible"=FALSE) -> ()  [unwired: 2 in, 2 out]
                n184 = property on="Ring" class="Ring (strict)"("Visible"=TRUE) -> ()  [unwired: 2 in, 2 out]
                n185 = Unbundle(w294) -> (w290:string[])
                n186 = Match First String(2:w290, 3:w295) -> (0:w291:i32)  [unwired: 1 out]
                n187 = property on="Ring" class="Ring (strict)"("Value"=w291, "Strings []"=w290) -> ()  [unwired: 2 in, 2 out]
              }
              frame "Exposure Priority  **" {
                n188 = call <vilib>:"NT Read String.vi"("Name"=w305) -> ("String"=w304:string)  [unwired: 9 in, 1 out]
                n189 = Index Array(array=w302, index=3) -> (element=w303:cluster{string[]})
                n190 = property on="Slider" class="Slide (strict)"("Visible"=FALSE) -> ()  [unwired: 2 in, 2 out]
                n191 = property on="Ring" class="Ring (strict)"("Visible"=TRUE) -> ()  [unwired: 2 in, 2 out]
                n192 = Unbundle(w303) -> (w299:string[])
                n193 = Match First String(2:w299, 3:w304) -> (0:w300:i32)  [unwired: 1 out]
                n194 = property on="Ring" class="Ring (strict)"("Value"=w300, "Strings []"=w299) -> ()  [unwired: 2 in, 2 out]
              }
              frame "Color Enable  **" {
                n195 = call <vilib>:"NT Read String.vi"("Name"=w314) -> ("String"=w313:string)  [unwired: 9 in, 1 out]
                n196 = Index Array(array=w311, index=4) -> (element=w312:cluster{string[]})
                n197 = property on="Slider" class="Slide (strict)"("Visible"=FALSE) -> ()  [unwired: 2 in, 2 out]
                n198 = property on="Ring" class="Ring (strict)"("Visible"=TRUE) -> ()  [unwired: 2 in, 2 out]
                n199 = Unbundle(w312) -> (w308:string[])
                n200 = Match First String(2:w308, 3:w313) -> (0:w309:i32)  [unwired: 1 out]
                n201 = property on="Ring" class="Ring (strict)"("Value"=w309, "Strings []"=w308) -> ()  [unwired: 2 in, 2 out]
              }
              frame Default {
                n202 = property on="Slider" class="Slide (strict)"("Visible"=FALSE) -> ()  [unwired: 2 in, 2 out]
                n203 = property on="Ring" class="Ring (strict)"("Visible"=FALSE) -> ()  [unwired: 2 in, 2 out]
              }
              frame "Brightness  **", "Color Level  **", "Compression  **", "FPS  **", "Sharpness  **" {
                n204 = call <vilib>:"NT Read Number.vi"("Name"=w320) -> ("Numeric"=w319:dbl)  [unwired: 9 in, 1 out]
                n205 = property on="Ring" class="Ring (strict)"("Visible"=FALSE) -> ()  [unwired: 2 in, 2 out]
                n206 = property on="Slider" class="Slide (strict)"("Visible"=TRUE, "Scale.Maximum"=100.0 ("Scale.Range:Maximum")) -> ()  [unwired: 2 in, 2 out]
                n207 = local write "Slider"(w319) -> ()
              }
            }
            n208 = property on="On/Off" class="Bool (strict)"("Visible"=FALSE) -> ()  [unwired: 2 in, 2 out]
            n209 = property on="Motor" class="Clust (strict)"("Visible"=FALSE) -> ()  [unwired: 2 in, 2 out]
          }
        }
      }
      event "Test Name": Mouse Enter {
        # "Populate the ring with the list of tests"
        n210 = event-data() -> ()  [unwired: 1 in, 1 out]
        n211 = call <vilib>:"NT Read String Array.vi"("Name"="TestMode/TestList") -> ("String Array"=w327:string[])  [unwired: 9 in, 1 out]
        n212 = Build Array (concatenate)("Select the test to run...", w327) -> (w326:string[])
        n213 = property on="Test Name" class="Ring (strict)"("Strings []"=w326) -> ()  [unwired: 2 in, 2 out]
      }
      event "Test Name": Value Change {
        w329 = FALSE ("Visible")
        # "Tell the robot the test name to run"
        n214 = event-data() -> ("NewVal"=w333:u16)  [unwired: 1 in]
        n215 = property on="Test Name" class="Ring (strict)"() -> ("Strings []"=w334:string[])  [unwired: 2 in, 2 out]
        n216 = property on="Ring" class="Ring (strict)"("Visible"=w329) -> ()  [unwired: 2 in, 2 out]
        n217 = property on="Motor" class="Clust (strict)"("Visible"=w329) -> ()  [unwired: 2 in, 2 out]
        n218 = property on="Slider" class="Slide (strict)"("Visible"=w329) -> ()  [unwired: 2 in, 2 out]
        n219 = property on="On/Off" class="Bool (strict)"("Visible"=w329) -> ()  [unwired: 2 in, 2 out]
        n220 = property on="Rev/Fwd" class="Clust (strict)"("Visible"=w329) -> ()  [unwired: 2 in, 2 out]
        n221 = local write "Progress"(T5 {"Test Progress"=0, "Test Progress Text"=""} ("Progress")) -> ()
        n222 = property on="Progress" class="Clust (strict)"("Visible"=TRUE) -> ()  [unwired: 2 in, 2 out]
        n223 = Index Array(array=w334, index=w333) -> (element=w332:string)
        n224 = call <vilib>:"NT Write String.vi"("String"=w332, "Name"="TestMode/TestName") -> ()  [unwired: 9 in, 1 out]
      }
      event "Listbox": Double Click {
        n225 = event-data() -> ("PlatMods.Shift"=w337:bool, "Row"=w339:i32)  [unwired: 1 in]
        n226 = case shown="False" w337 {
          tunnel: w339 -> [w343 _]
          tunnel: 1 -> [w342 _]
          frame False {
            n227 = property on="Listbox" class="LstBox (strict)"() -> ("Item Symbols"=w341:i32[])  [unwired: 2 in, 2 out]
            n228 = Replace Array Subset(array=w341, new element=w342, index=w343) -> (w340:i32[])
            n229 = property on="Listbox" class="LstBox (strict)"("Item Symbols"=w340) -> ()  [unwired: 2 in, 2 out]
          }
          frame True {
            w344 = 0 ("Top Row")
            n230 = property on="Listbox" class="LstBox (strict)"() -> ("Number of Rows"=w346:u32)  [unwired: 2 in, 2 out]
            n231 = Initialize Array(0, w346) -> (w345:i32[])
            n232 = property on="Listbox" class="LstBox (strict)"("Top Row"=w344, "Value"=w344, "Item Symbols"=w345) -> ()  [unwired: 2 in, 2 out]
          }
        }
      }
      event "Listbox": Key Down {
        n233 = event-data() -> ("VKey"=w350:T16)  [unwired: 1 in]
        n234 = case shown="\"Left\", \"Right\"" w350 {
          selector: w350 -> [w355 _]
          tunnel: eventvkey."Left" ("VKey") -> [w353 _]
          frame "Left", "Right" {
            n235 = Equal?(x=w353, y=w355) -> (x = y?=w354:bool)
            n236 = Select(t=0, s=w354, f=1) -> (s? t:f=w356:i32)
            n237 = property on="Listbox" class="LstBox (strict)"() -> ("Item Symbols"=w359:i32[])  [unwired: 2 in, 2 out]
            n238 = Replace Array Subset(array=w359, new element=w356, index="Listbox") -> (w358:i32[])
            n239 = property on="Listbox" class="LstBox (strict)"("Item Symbols"=w358) -> ()  [unwired: 2 in, 2 out]
          }
          frame Default {
          }
        }
      }
      event "DB Camera Config": Value Change {
        n240 = event-data() -> ("NewVal"=w363:bool)  [unwired: 1 in]
        n241 = case shown="False" w363 {
          tunnel: w362 -> [w372 _]
          tunnel: [w365 w383] -> w361
          tunnel: w360 -> [w364 w383]
          frame False {
            w379 = "Camera"
            w382 = FALSE ("Visible")
            n242 = property on="Camera Settings" class="Clust (strict)"("Visible"=w382) -> ()  [unwired: 2 in, 2 out]
            n243 = local write "DB Camera Config"(w382) -> ()
            n244 = local read "Camera Settings"() -> (w371:T1)
            n245 = Index Array(array=w372) -> (element=w375:cluster{string[]})  [unwired: 1 in]
            n246 = Unbundle(w375) -> (w374:string[])
            n247 = Unbundle(w371) -> ("Frate Rate"=w370:i32, "Compression"=w369:i32, "Size"=w373:u16)
            n248 = Index Array(array=w374, index=w373) -> (element=w368:string)
            n249 = call-poly <vilib>:"Write Key.vi"("section"=w379, "value"=w368, "key"="Size", "refnum"=w364) -> ("refnum out"=w381:T15)  [unwired: 2 in, 5 out]
            n250 = call-poly <vilib>:"Write Key.vi"("section"=w379, "value"=w370, "key"="FrameRate", "refnum"=w381) -> ("refnum out"=w380:T15)  [unwired: 1 in, 6 out]
            n251 = call-poly <vilib>:"Write Key.vi"("section"=w379, "value"=w369, "key"="Compression", "refnum"=w380) -> ("refnum out"=w366:T15)  [unwired: 1 in, 6 out]
            n252 = call <vilib>:"Close Config Data.vi"("refnum"=w366) -> ("file path"=w367:path)  [unwired: 2 in, 8 out]
            n253 = call <vilib>:"Open Config Data.vi"("configuration file path"=w367) -> ("refnum"=w365:T15)  [unwired: 8 in, 2 out]
          }
          frame True {
            n254 = property on="Camera Settings" class="Clust (strict)"("Visible"=TRUE) -> ()  [unwired: 2 in, 2 out]
          }
        }
      }
      event "Camera Settings": Value Change {
        n255 = event-data() -> ("NewVal"=w396:T1)  [unwired: 1 in]
        n256 = Index Array(array=w392) -> (element=w391:cluster{string[]})  [unwired: 1 in]
        n257 = Unbundle(w391) -> (w390:string[])
        n258 = Unbundle(w396) -> ("Frate Rate"=w387:i32, "Compression"=w386:i32, "Size"=w389:u16)
        n259 = Index Array(array=w390, index=w389) -> (element=w388:string)
        n260 = Format Into String(format string="%s   %dfps   %d%%", w388, w387, w386) -> (resulting string=w393:string)  [unwired: 2 in, 1 out]
        n261 = Build Array(w393) -> (w394:string[])
        n262 = property on="DB Camera Config" class="Bool (strict)"("Strings [4]"=w394) -> ()  [unwired: 2 in, 2 out]
      }
      event "Motor.Enable": Value Change {
        n263 = event-data() -> ("NewVal"=w402:bool)  [unwired: 1 in]
        n264 = Unbundle("Motor") -> ("Value"=w401:dbl)  [unwired: 1 out]
        n265 = Select(t=w401, s=w402, f=0.0) -> (s? t:f=w399:dbl)
        n266 = call <vilib>:"NT Write Number.vi"("Numeric"=w399, "Name"=w398) -> ()  [unwired: 9 in, 1 out]
      }
      event "Slider": Value Change {
        n267 = event-data() -> ("NewVal"=w405:dbl)  [unwired: 1 in]
        n268 = call <vilib>:"NT Write Number.vi"("Numeric"=w405, "Name"=w406) -> ()  [unwired: 9 in, 1 out]
      }
      event "On/Off": Value Change {
        n269 = event-data() -> ("NewVal"=w410:bool)  [unwired: 1 in]
        n270 = Boolean To (0,1)(Boolean=w410) -> (0, 1=w409:i16)
        n271 = call <vilib>:"NT Write Number.vi"("Numeric"=w409, "Name"=w408) -> ()  [unwired: 9 in, 1 out]
      }
      event "Rev/Fwd": Value Change {
        n272 = event-data() -> ("NewVal.Forward"=w418:bool, "NewVal.Reverse"=w417:bool)  [unwired: 1 in]
        n273 = Boolean To (0,1)(Boolean=w417) -> (0, 1=w416:i16)
        n274 = Boolean To (0,1)(Boolean=w418) -> (0, 1=w414:i16)
        n275 = Negate(x=w416) -> (-x=w415:i16)
        n276 = Add(x=w414, y=w415) -> (x+y=w413:i16)
        n277 = call <vilib>:"NT Write Number.vi"("Numeric"=w413, "Name"=w412) -> ()  [unwired: 9 in, 1 out]
      }
      event "Ring": Value Change {
        n278 = event-data() -> ("NewVal"=w422:u16)  [unwired: 1 in]
        n279 = property on="Ring" class="Ring (strict)"() -> ("Strings []"=w423:string[])  [unwired: 2 in, 2 out]
        n280 = Index Array(array=w423, index=w422) -> (element=w421:string)
        n281 = call <vilib>:"NT Write String.vi"("String"=w421, "Name"=w420) -> ()  [unwired: 9 in, 1 out]
      }
    }
  }
  n282 = property on="Camera Settings" class="Clust (strict)"("Val(Sgnl)"=w4) -> ()  [unwired: 2 in, 2 out]
